vi "triangle_source.vi"(2 "protect_scan":bool, 3 "pause":bool, 4 "triangle_control":T1 {"end_source / V" format="%#_13g"; "lower_volt_limit / V" format="%#_13g"; "upper_volt_limit / V" format="%#_13g"; "step_voltage / V" format="%#_13g"; "init_source / V" format="%#_13g"}) -> (0 "terminate?":bool, 1 "output_signal / V":dbl format="%#_13g")   [LabVIEW 2014]
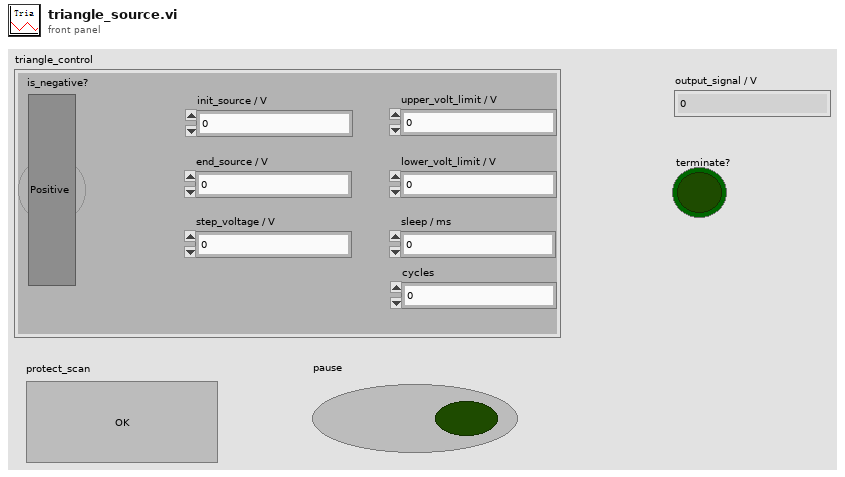
[diagram p1: front panel]
types:
  T1 = cluster{"init_source / V":dbl, "step_voltage / V":dbl, "upper_volt_limit / V":dbl, "lower_volt_limit / V":dbl, "sleep / ms":u32, "is_negative?":bool, "cycles":u32, "end_source / V":dbl}
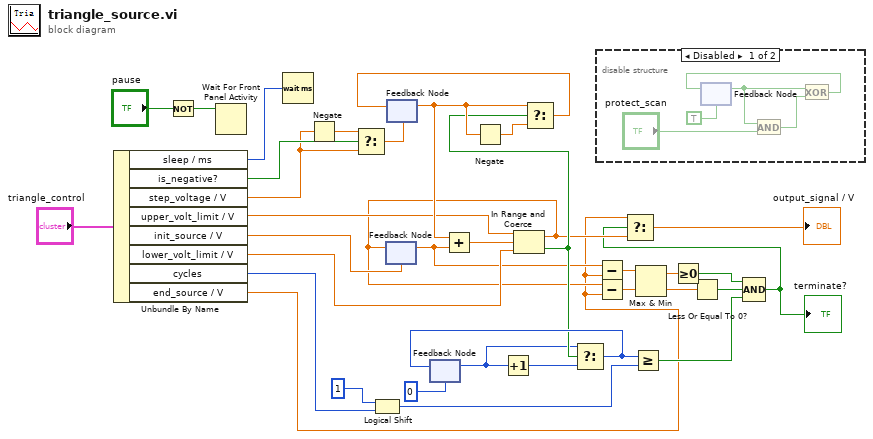
[diagram p0: block diagram]
diagram:
  n1 = Unbundle By Name("triangle_control") -> ("sleep / ms"=w29:u32, "is_negative?"=w28:bool, "step_voltage / V"=w27:dbl, "upper_volt_limit / V"=w26:dbl, "init_source / V"=w25:dbl, "lower_volt_limit / V"=w24:dbl, "cycles"=w22:u32, "end_source / V"=w4:dbl)
  n2 = Not(x="pause") -> (.not. x?=w5:bool)
  n3 = Wait For Front Panel Activity(3:w5) -> ()  [unwired: 2 in, 1 out]
  n4 = Wait (ms)(milliseconds to wait=w29) -> ()  [unwired: 1 out]
  n5 = Negate(x=w27) -> (-x=w34:dbl)
  n6 = Select(t=w34, s=w28, f=w27) -> (s? t:f=w35:dbl)
  n7 = Logical Shift(y=i16 1, x=w22) -> (x << y=w20:u32)
  n8 = feedback #1(w25) -> (w16:dbl)
  n9 = feedback #2(w35) -> (w33:dbl)
  n10 = feedback #3(0) -> (w2:i32)
  n11 = Add(x=w33, y=w16) -> (x+y=w17:dbl)
  n12 = Negate(x=w33) -> (-x=w32:dbl)
  n13 = Increment(x=w2) -> (x+1=w1:i32)
  n14 = In Range and Coerce(upper limit=w26, x=w17, lower limit=w24) -> (coerced(x)=w7:dbl, In Range?=w18:bool)
  n15 = feedback-in #1(w7) -> ()
  n16 = Select(t=w33, s=w18, f=w32) -> (s? t:f=w31:dbl)
  n17 = feedback-in #2(w31) -> ()
  n18 = Select(t=w2, s=w18, f=w1) -> (s? t:f=w19:i32)
  n19 = feedback-in #3(w19) -> ()
  n20 = disable-structure shown="Disabled" {
    frame Disabled {
      n21 = feedback #4(TRUE) -> (w38:bool)
      n22 = And(x=w38, y="protect_scan") -> (x .and. y?=w36:bool)
      n23 = Exclusive Or(1:w36, 2:w38) -> (0:w37:bool)
      n24 = feedback-in #4(w37) -> ()
    }
    frame Enabled {
    }
  }
  n25 = Subtract(x=w16, y=w4) -> (x-y=w15:dbl)
  n26 = Subtract(x=w7, y=w4) -> (x-y=w14:dbl)
  n27 = Greater Or Equal?(x=w19, y=w20) -> (x >= y?=w9:bool)
  n28 = Max & Min(x=w15, y=w14) -> (max(x,y)=w13:dbl, min(x,y)=w12:dbl)
  n29 = Greater Or Equal To 0?(x=w13) -> (x >= 0?=w11:bool)
  n30 = Less Or Equal To 0?(x=w12) -> (x <= 0?=w10:bool)
  n31 = Compound Arithmetic op=AND(w11, w10, w9) -> (w3:bool)
  "terminate?" <- w3
  n32 = Select(t=w4, s=w3, f=w7) -> (s? t:f=→"output_signal / V":dbl)
